vi "IO20 SendCmd.vi"(8 "error in":errorcluster, 10 "CMD":T1=enum."LED ON", 11 "IO20 VISA":refnum<visa-resource-name>) -> (0 "error out":errorcluster, 1 "ADC Data Out":cluster{"DAQ Channel":string, "ADC Voltage":dbl}, 2 "ADC Voltage":dbl, 3 "IO20 VISA-OUT":refnum<visa-resource-name>, 5 "ADC Volt":bool, 7 "Read Buffer":string)   [LabVIEW 2020, in "DLP Design Modules Driver.lvlib"]
doc: "With the CMD typedef [IO20_Config1_typedef.ctl] definition the ports on the IO20 device are configured as follows,\n\n- P5, P6, and P7 are configured as Digital Outputs, Hi = 1.2V (at least on my dev board), Lo = 0V\n\n- RB6, RB7, AN0, AN1, and AN2 are configured as Digital Inputs\n\n- AN3 through AN13 are configured as analog inputs (10 bit resolution, 5V referenced from USB bus)\n\nThe CMD typedef also allows full control of the two on-board SPDT relays and full control of the on-board LED."
uses:
  DLP Design Modules Driver.lvlib
  IO20_Config1_typedef.ctl
  <vilib>/Instr/_visa.llb/VISA Configure Serial Port (Instr).vi
panel:
  out "MSB LSB":string
  out "ADC Counts":i16
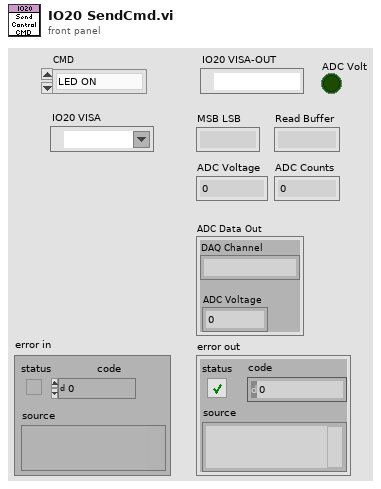
[diagram p1: front panel]
types:
  T1 = typedef "DLP Design Modules Driver.lvlib/IO20_Config1_typedef.ctl" = enum16{"Ping", "Flash LED", "LED OFF", "LED ON", "Relay 1 Set", "Relay 1 Reset", "Relay 2 Set", "Relay 2 Reset", "AN0-DI", "AN1-DI", "AN2-DI", "RB6-DI", "RB7-DI", "AN3-AI", "AN4-AI", "AN5-AI", "AN6-AI", "AN7-AI", "AN8-AI", "AN9-AI", "AN10-AI", "AN11-AI", "AN12-AI", "AN13-AI", "P5-DO-low", "P5-DO-high", "P6-DO-low", "P6-DO-high", "P7-DO-low", "P7-DO-high"}
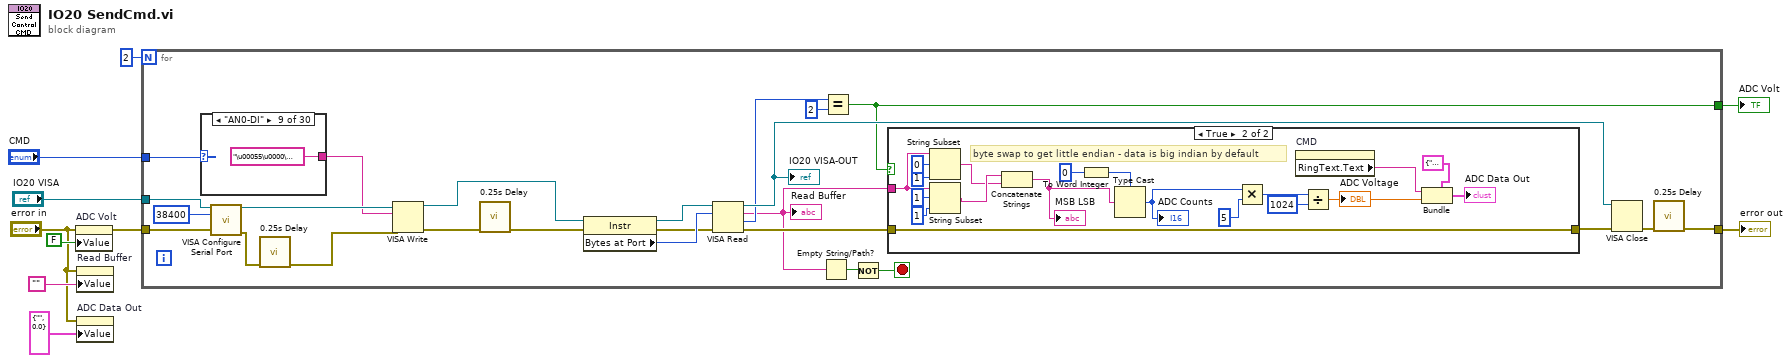
[diagram p0: block diagram]
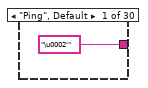
[diagram p2: hidden frame]
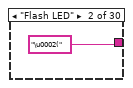
[diagram p3: hidden frame]
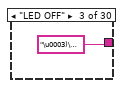
[diagram p4: hidden frame]
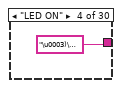
[diagram p5: hidden frame]
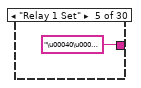
[diagram p6: hidden frame]
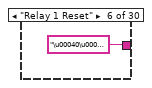
[diagram p7: hidden frame]
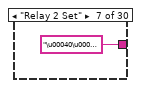
[diagram p8: hidden frame]
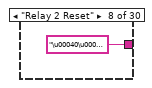
[diagram p9: hidden frame]
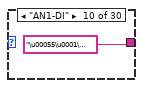
[diagram p10: hidden frame]
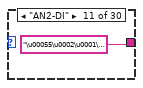
[diagram p11: hidden frame]
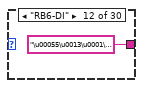
[diagram p12: hidden frame]
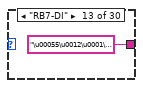
[diagram p13: hidden frame]
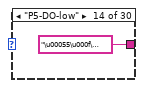
[diagram p14: hidden frame]
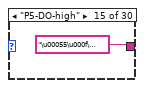
[diagram p15: hidden frame]
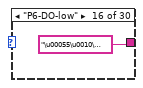
[diagram p16: hidden frame]
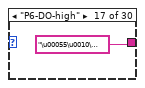
[diagram p17: hidden frame]
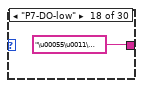
[diagram p18: hidden frame]
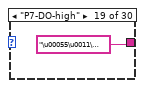
[diagram p19: hidden frame]
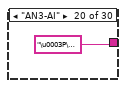
[diagram p20: hidden frame]
diagram:
  n1 = property on="ADC Volt" class="Bool (strict)"(error in="error in", "Value"=FALSE ("Read")) -> (error out=w9:errorcluster)  [unwired: 1 in, 1 out]
  n2 = property on="Read Buffer" class="Str"(error in="error in", "Value"="") -> ()  [unwired: 1 in, 2 out]
  n3 = property on="ADC Data Out" class="Clust (strict)"(error in="error in", "Value"=cluster{"RingText.Text":string, dbl} {"RingText.Text"="", 0.0} ("ADC Data")) -> ()  [unwired: 1 in, 2 out]
  n4 = for {
    N: 2 -> [_]
    tunnel: w9 -> [w22]
    tunnel: [w24] -> w3
    tunnel: [w26] -> w8
    tunnel: "IO20 VISA" -> [w21]
    tunnel: "CMD" -> [w15]
    stop <- w11 stop-if-true
    n5 = case shown="\"AN0-DI\"" w15 {
      tunnel: ["\u0002'" ("write buffer") "\u0002(" ("write buffer") "\u0003)\u0001" ("write buffer") "\u0003)\u0000" ("write buffer") "\u00040\u0001\u0000" ("write buffer") "\u00040\u0001\u0001" ("write buffer") "\u00040\u0002\u0000" ("write buffer") "\u00040\u0002\u0001" ("write buffer") "\u00055\u0000\u0001\u0000" ("write buffer") "\u00055\u0001\u0001\u0000" ("write buffer") "\u00055\u0002\u0001\u0000" ("write buffer") "\u00055\u0013\u0001\u0000" ("write buffer") "\u00055\u0012\u0001\u0000" ("write buffer") "\u00055\u000f\u0000\u0000" ("write buffer") "\u00055\u000f\u0000\u0001" ("write buffer") "\u00055\u0010\u0000\u0000" ("write buffer") "\u00055\u0010\u0000\u0001" ("write buffer") "\u00055\u0011\u0000\u0000" ("write buffer") "\u00055\u0011\u0000\u0001" ("write buffer") "\u0003P\u0003" ("write buffer") "\u0003P\u0004" ("write buffer") "\u0003P\u0005" ("write buffer") "\u0003P\u0006" ("write buffer") "\u0003P\u0007" ("write buffer") "\u0003P\b" ("write buffer") "\u0003P\t" ("write buffer") "\u0003P\n" ("write buffer") "\u0003P\u000b" ("write buffer") "\u0003P\f" ("write buffer") "\u0003P\r" ("write buffer")] -> w14
      frame "Ping", Default {
      }
      frame "Flash LED" {
      }
      frame "LED OFF" {
      }
      frame "LED ON" {
      }
      frame "Relay 1 Set" {
      }
      frame "Relay 1 Reset" {
      }
      frame "Relay 2 Set" {
      }
      frame "Relay 2 Reset" {
      }
      frame "AN0-DI" {
      }
      frame "AN1-DI" {
      }
      frame "AN2-DI" {
      }
      frame "RB6-DI" {
      }
      frame "RB7-DI" {
      }
      frame "P5-DO-low" {
      }
      frame "P5-DO-high" {
      }
      frame "P6-DO-low" {
      }
      frame "P6-DO-high" {
      }
      frame "P7-DO-low" {
      }
      frame "P7-DO-high" {
      }
      frame "AN3-AI" {
      }
      frame "AN4-AI" {
      }
      frame "AN5-AI" {
      }
      frame "AN6-AI" {
      }
      frame "AN7-AI" {
      }
      frame "AN8-AI" {
      }
      frame "AN9-AI" {
      }
      frame "AN10-AI" {
      }
      frame "AN11-AI" {
      }
      frame "AN12-AI" {
      }
      frame "AN13-AI" {
      }
    }
    n6 = call-poly "VISA Configure Serial Port"("VISA resource name"=w21, "baud rate (9600)"=u32 38400, "error in (no error)"=w22) -> ("VISA resource name out"=w16:refnum<visa-resource-name>, "error out"=w20:errorcluster)  [unwired: 11 in]
    n7 = call "0.25s Delay"("error in (no error)"=w20) -> ("error out"=w17:errorcluster)  [unwired: 10 in]
    n8 = VISA Write(VISA resource name=w16, write buffer=w14, error in (no error)=w17) -> (VISA resource name out=w18:refnum<visa-resource-name>, error out=w19:errorcluster)  [unwired: 1 out]
    n9 = call "0.25s Delay"("error in (no error)"=w19) -> ("error out"=w35:errorcluster)  [unwired: 10 in]
    n10 = property class="Instr"(reference=w18, error in=w35) -> (reference out=w31:refnum<visa-resource-name>, error out=w29:errorcluster, "Bytes at Port"=w30:u32)
    n11 = VISA Read(VISA resource name=w31, byte count=w30, error in (no error)=w29) -> (VISA resource name out=w34:refnum<visa-resource-name>, read buffer=w13:string, return count=w33:u32, error out=w28:errorcluster)
    "Read Buffer" <- w13
    "IO20 VISA-OUT" <- w34
    n12 = Empty String/Path?(string/path=w13) -> (empty?=w12:bool)
    n13 = Equal?(x=w33, y=u32 2) -> (x = y?=w26:bool)
    n14 = Not(x=w12) -> (.not. x?=w11:bool)
    n15 = case shown="True" w26 {
      tunnel: w13 -> [_ w77]
      tunnel: w28 -> [w66 w79]
      tunnel: [w66 w79] -> w27
      frame False {
      }
      frame True {
        # "byte swap to get little endian - data is big indian by default"
        n16 = String Subset(string=w77, offset (0)=0 ("number"), length (rest)=1 ("number")) -> (substring=w71:string)
        n17 = String Subset(string=w77, offset (0)=1 ("number"), length (rest)=1 ("number")) -> (substring=w72:string)
        n18 = Concatenate Strings(w72, w71) -> (w83:string)
        "MSB LSB" <- w83
        n19 = To Word Integer(number=0) -> (16bit integer=w82:i16)
        n20 = Type Cast(type=w82, x=w83) -> (*(type *) &x=w84:i16)
        "ADC Counts" <- w84
        n21 = Multiply(x=w84, y=i16 5) -> (x*y=w85:i16)
        n22 = property on="CMD" class="Enum (strict)"() -> ("RingText.Text"=w69:string)  [unwired: 2 in, 2 out]
        n23 = Divide(x=w85, y=i16 1024) -> (x/y=w70:dbl)
        "ADC Voltage" <- w70
        n24 = Bundle(cluster=cluster{"RingText.Text":string, dbl} {"RingText.Text"="", 0.0}, "RingText.Text"=w69, w70) -> (→"ADC Data Out":cluster{"RingText.Text":string, dbl})
      }
    }
    n25 = VISA Close(VISA resource name=w34, error in (no error)=w27) -> (error out=w25:errorcluster)
    n26 = call "0.25s Delay"("error in (no error)"=w25) -> ("error out"=w24:errorcluster)  [unwired: 10 in]
  }
  "error out" <- w3
  "ADC Volt" <- w8
